vi "Set Inspection Relative [FLR].vi"(7 "Micropulse # In":i32, 8 "error in (no error)":errorcluster, 9 "Direction":T1, 10 "End Location (mm)":dbl=1.0 min=1.0 max=100000.0, 11 "Axis No.":u8=1 min=1 max=4) -> (0 "error out":errorcluster, 5 "Micropulse # Out":i32)   [LabVIEW 2026, in "MicroPulse_Driver.lvlib"]
doc: "To enable FLR mode for a relative displacement.\n\nFormat:\nFLR <axis><displacement><direction>\n\nDescription:\nFLR inspection mode is enabled. Inspection begins at the current location and continues at each subsequent SPA point reached in the specified direction (0 = forwards, 1 = backwards) until the axis has moved the specified displacement. LCP commands may be used during the inspection and will not affect the displacement calculations. At the end of the displacement the MSE command line is invoked.\n\nParameters:\n<axis> : axis number 1 to 4\n\n<displacement> : Relative displacement in distance units 0 to 1600000000. If a distance of 0 is specified, then the inspection will be performed in the direction specified without an end point. In this instance care should be taken to ensure the 32bit encoders stay below within the valid range.\n\n<direction> :\n0 = Inspect forward\n1 = Inspect backwards\n2 = Inspect in both directions continually (ignoring any set BKL timeout) until the mode is exited. When 2 is used set the displacement to zero.\n\nExample:\nFLR 2 100 1 : Inspect on axis 2 for 100 distance (SPA) units in a negative direction"
uses:
  MicroPulse_Driver.lvlib
  Data/Datatypes/MP - inspection direction (relative).ctl
  Private/MP-Registry Action-Enum.ctl
  <instrlib>/Micropulse/Micropulse.lvlib
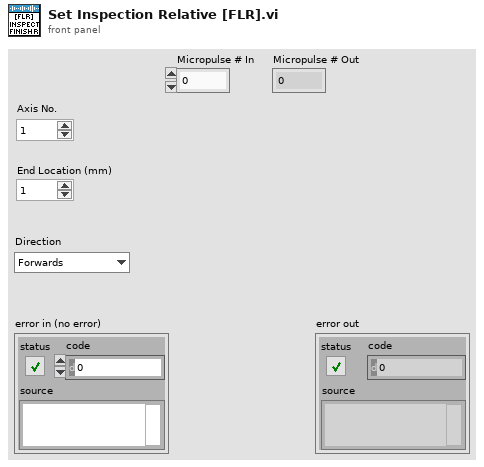
[diagram p1: front panel]
types:
  T1 = typedef "Micropulse.lvlib/MP - inspection direction (relative).ctl" = enum16{"Forwards", "Backwards", "Bidirectional"}
  T2 = typedef "MicroPulse_Driver.lvlib/MP-Registry Action-Enum.ctl" = enum16{"Read", "Add Test", "Add Command", "Add Gate Command", "Add Encoder Command", "Clear Command  List", "Set Registry", "Set System Details", "Set DOF", "Set Velocity", "Disable Asynch Reads", "Enable Asynch Reads", "Add Connection", "Disconnect", "Shutdown"}
  T3 = typedef "Micropulse.lvlib/MP-Registry Data-Cluster.ctl" = cluster{"Instrument Type":T4, "Serial #":u64, "Sample Frequency":T5, "dt (us)":dbl, "DOF":T6, "Material Velocity":dbl, "Asynch Reads":T7, "NUM of Tests":u32, "System Details":T8, "Gates":T10[], "Encoders":T17[], "CMD LUT":variant, "Command List":string}
  T4 = typedef "Micropulse.lvlib/MP - instrument type.ctl" = enum16{"MicroPulse 5", "LT1", "LT2", "LTPA", "MPLT", "MicroPulse 6", "PipeScanner", "<MicroPulse>", "Micropulse 4", "Simulated Data"}
  T5 = typedef "Micropulse.lvlib/MP - sample frequency.ctl" = enum16{"Use Default", "200MHz (LT2 only)", "100MHz", "50MHz", "25MHz", "10MHz"}
  T6 = typedef "Micropulse.lvlib/MP - data output format.ctl" = enum16{"", "8-bit Mode", "10-bit Mode", "12-bit Mode", "16-bit Mode", "8-bit Log Mode", "12-bit Packed Mode"}
  T7 = typedef "Micropulse.lvlib/MP - asynch read mode.ctl" = enum16{"Disabled", "Enabled"}
  T8 = typedef "Micropulse.lvlib/MP - general system status.ctl" = cluster{"System Type":T4, "Serial No.":u64, "Channels":cluster{"Conv":u8, "PA":u16, "Extra":u32}, "Sample Frequency":cluster{"Default":u8, "Actual":u8}, "Software Versions":string, "Data Output Format":cluster{"Default":T6, "Actual":T6}, "Temperatures":cluster{"System":u8, "Processor":u8, "Slave Sys":u8, "Slave Proc":u8}, "Tx Buffer Size":u32, "System Error":string, "No. of Cards":u8, "DAC Gain":i16, "Uptimes":cluster{"since Power":u32, "since RSTS":u32, "since SRST":u32}, "Voltages":cluster{"Nominal":dbl, "Measured":dbl, "Difference":dbl}[], "Interface Cards":T9[]}
  T9 = typedef "Micropulse.lvlib/MP - interface card status.ctl" = cluster{"Status":u8, "Map":u8, "Board - T":u8, "FPGA - T":u8, "PAIF Status":string, "Version":string}
  T10 = typedef "Micropulse.lvlib/MP - Registry Gates.ctl" = cluster{"Display Gate":T11, "ETM Mode":T12, "Echo Gate":T13, "Insp Gates":T14[]}
  T11 = typedef "Micropulse.lvlib/MP - display gate.ctl" = cluster{"Start":dbl, "Length":dbl}
  T12 = typedef "Micropulse.lvlib/MP - echo gate mode.ctl" = enum16{"Echo Trigger OFF", "Echo Gate Display Mode", "Echo Trigger ON", "Multi Gate or FMC Mode", "Reserved", "PA - Echo Trigger ON"}
  T13 = typedef "Micropulse.lvlib/MP - echo gate parameters.ctl" = cluster{"Start (us)":dbl, "Length (us)":dbl, "Threshold":u16, "Colour":u32}
  T14 = typedef "Micropulse.lvlib/MP - multigate inspection gate parameters.ctl" = cluster{"Start (us)":dbl, "Length (us)":dbl, "Threshold":u16, "Enabled?":bool, "Max # Peaks":u16, "Hysteresis":T15, "Mode":T16, "Inverted?":bool, "Colour ":u32}
  T15 = typedef "Micropulse.lvlib/MP - hysteresis level.ctl" = enum16{"None", "3dB", "6dB", "9dB", "12dB"}
  T16 = typedef "Micropulse.lvlib/MP - multigate mode.ctl" = enum16{"1st Peak in Gate", "Largest Peak In Gate", "All Peaks In Gate", "1st Threshold Crossing"}
  T17 = typedef "Micropulse.lvlib/MP - encoder settings.ctl" = cluster{"Encoder Type":T18, "Counts/mm":u32, "Enable Termination?":bool, "Multiplier":u32, "Backlash Period (s)":dbl, "Encoder Filter":u32}
  T18 = typedef "Micropulse.lvlib/MP - encoder type.ctl" = enum16{"Quadrature", "Step/Direction"}
  T19 = typedef "Micropulse.lvlib/TCP config.ctl" = cluster{"Connection ID":refnum<k5>, "IP address":string, "host port":u16, "OC timeout":i32, "Read timeout":i32, "Write timeout":i32}
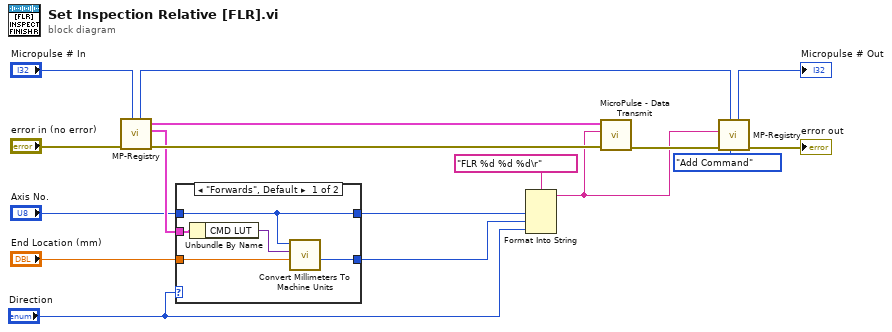
[diagram p0: block diagram]
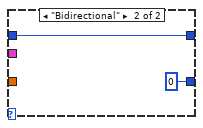
[diagram p2: hidden frame]
diagram:
  n1 = call "MP-Registry.vi"("Micropulse # In"="Micropulse # In", "error in (no error)"="error in (no error)") -> ("error out"=w15:errorcluster, "Micropulse Data"=w6:T3, "TCP config"=w14:T19, "Micropulse # Out"=w11:i32)  [unwired: 6 in]
  n2 = case shown="\"Forwards\", Default" "Direction" {
    tunnel: w6 -> [w22 _]
    tunnel: "Axis No." -> [w18 w23]
    tunnel: "End Location (mm)" -> [w20 _]
    tunnel: [w19 u32 0 ("Distance (MU)")] -> w4
    tunnel: [w18 w23] -> w1
    frame "Forwards", Default {
      n3 = Unbundle By Name(w22) -> ("CMD LUT"=w21:variant)
      n4 = call "Convert Millimeters To Machine Units.vi"("Distance (mm)"=w20, "CMD LUT"=w21, "Axis No."=w18) -> ("Distance (MU)"=w19:u32)  [unwired: 8 in]
    }
    frame "Bidirectional" {
    }
  }
  n5 = Format Into String(format string="FLR %d %d %d\r", w1, w4, "Direction") -> (resulting string=w8:string)  [unwired: 2 in, 1 out]
  n6 = call "MicroPulse - Data Transmit.vi"("error in (no error)"=w15, "data"=w8, "TCP config"=w14) -> ("error out"=w12:errorcluster)  [unwired: 6 in, 2 out]
  n7 = call "MP-Registry.vi"("Action"=MP-Registry_Action-Enum."Add Command", "Micropulse # In"=w11, "error in (no error)"=w12, "Data in"=w8) -> ("error out"=→"error out":errorcluster, "Micropulse # Out"=→"Micropulse # Out":i32)  [unwired: 4 in, 2 out]
